vi "Cycle_Time_Test.vi"() -> ()   [LabVIEW 2017]
uses:
  Controls/ADCP_UI/ADCP_UI_Data_Packet_Receiver_Parameters.ctl
  Controls/Connection Management/Connection_Management_Commands.ctl
  Controls/Packet/Packet.ctl
  Controls/Packet/Packet_Direction.ctl
  Controls/Packet/Packet_Type.ctl
  Controls/Packet/Packet_Priority.ctl
  <vilib>/Instr/_visa.llb/VISA Flush IO Buffer Mask.ctl
panel:
  in  "Node ID":u8
  in  "Stop":bool
  out "Received Packet Data":T1[](array[typedef])
  in  "baud rate":u32=9600
  in  "COM Port In":refnum<visa-resource-name>
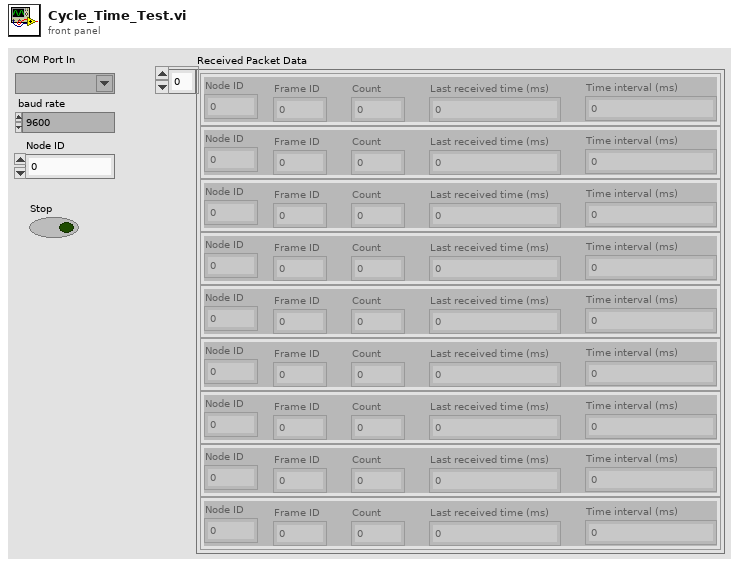
[diagram p1: front panel]
types:
  T1 = typedef "ADCP_UI_Data_Packet_Receiver_Parameters.ctl" = cluster{"Node ID":u32, "Frame ID":u32, "Count":u32, "Last received time (ms)":u32, "Time interval (ms)":u32}
  T2 = typedef "Packet.ctl" = cluster{"Raw Bytes":u8[], "Checksum":bool, "Direction":T3, "Processed Bytes":u8[], "Node ID":u8, "Packet type":T4, "Frame Data":u32, "Priority":T5, "Frame ID":u8}
  T3 = typedef "Packet_Direction.ctl" = enum16{"Transmit", "Receive", "Bidirectional"}
  T4 = typedef "Packet_Type.ctl" = enum16{"Data", "Connection Management", "Remote Request", "Error/Status"}
  T5 = typedef "Packet_Priority.ctl" = enum16{"LOW", "HIGH"}
  T6 = typedef "Connection_Management_Commands.ctl" = enum16{"Sync/Reset", "Open Connection", "Close Connection"}
  T7 = typedef "VISA Flush IO Buffer Mask.ctl" = u16
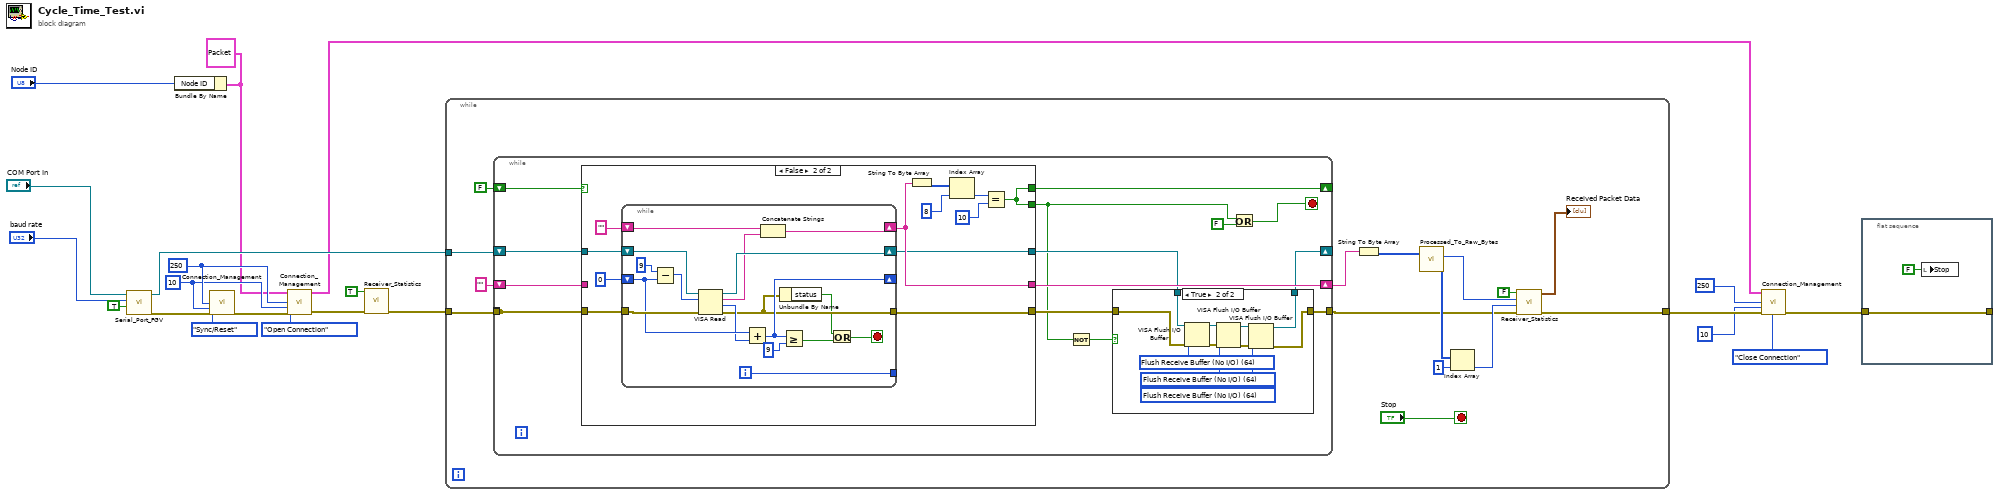
[diagram p0: block diagram]
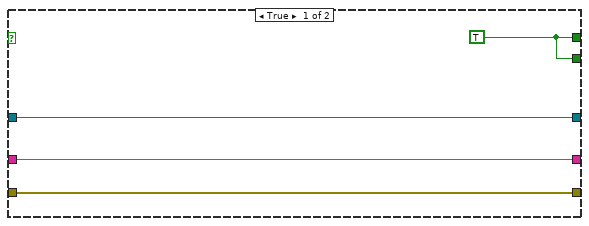
[diagram p3: hidden frame]
diagram:
  w3 = T2 {"Raw Bytes"=[], "Checksum"=FALSE, "Direction"=enum."Transmit", "Processed Bytes"=[], "Node ID"=0, "Packet type"=enum."Data", "Frame Data"=0, "Priority"=enum."LOW", "Frame ID"=0} ("CM Packet In")
  w14 = u8 10 ("Number of tries")
  w15 = 250 ("Retry interval (ms)")
  n1 = call "Serial_Port_FGV.vi"("Initialize ?"=TRUE, "baud rate"="baud rate", "COM Port In"="COM Port In") -> ("error out"=w18:errorcluster, "COM Port out"=w12:refnum<visa-resource-name>)  [unwired: 7 in]
  n2 = Bundle By Name(cluster=w3, "Node ID"="Node ID") -> ()  [unwired: 1 out]
  n3 = call "Connection_Management.vi"("Commands"=Connection_Management_Commands."Sync/Reset", "Retry interval (ms)"=w15, "Number of tries"=w14, "error in (no error)"=w18) -> ("error out"=w16:errorcluster)  [unwired: 8 in, 3 out]
  n4 = call "Connection_Management.vi"("CM Packet In"=w3, "Commands"=Connection_Management_Commands."Open Connection", "Retry interval (ms)"=w15, "Number of tries"=w14, "error in (no error)"=w16) -> ("CM Packet Out"=w1:T2, "error out"=w5:errorcluster)  [unwired: 7 in, 2 out]
  n5 = call "Receiver_Statistics.vi"("error in (no error)"=w5, "Initialize ?"=TRUE) -> ("error out"=w4:errorcluster)  [unwired: 7 in, 2 out]
  n6 = while {
    tunnel: w12 -> [w34]
    tunnel: w4 -> [w33]
    tunnel: [w22] -> w10
    stop <- "Stop" stop-if-true
    n7 = while {
      tunnel: w33 -> [w45]
      shift-right: [w48] -> _
      shift-left: FALSE -> [w49]
      tunnel: [w43] -> w23
      shift-right: [w47] -> w31
      shift-left: "" -> [w46]
      shift-right: [w41] -> _
      shift-left: w34 -> [w50]
      tunnel: [w45] -> _
      stop <- w40 stop-if-true
      n8 = case shown="False" w49 {
        tunnel: w45 -> [w66 w79]
        tunnel: w50 -> [w64 w77]
        tunnel: [w67 w71] -> w38
        tunnel: [w67 w71] -> w48
        tunnel: [w66 w70] -> w44
        tunnel: [w65 w69] -> w47
        tunnel: w46 -> [w65 _]
        tunnel: [w64 w68] -> w42
        frame True {
          w67 = TRUE
        }
        frame False {
          n9 = while {
            tunnel: w79 -> [w96]
            shift-right: [w86] -> _
            shift-left: 0 -> [w89]
            shift-right: [w92] -> w68
            shift-left: w77 -> [w93]
            shift-right: [w85] -> w69
            shift-left: "" -> [w91]
            tunnel: [w81] -> w70
            tunnel: [w84] -> _
            i -> [w84]
            stop <- w83 stop-if-true
            n10 = Subtract(x=9, y=w89) -> (x-y=w94:u32)
            n11 = VISA Read(VISA resource name=w93, byte count=w94, error in (no error)=w96) -> (VISA resource name out=w92:refnum<visa-resource-name>, read buffer=w90:string, return count=w88:u32, error out=w81:errorcluster)
            n12 = Add(x=w89, y=w88) -> (x+y=w86:u32)
            n13 = Concatenate Strings(w91, w90) -> (w85:string)
            n14 = Unbundle By Name(w81) -> ("status"=w80:bool)
            n15 = Greater Or Equal?(x=w86, y=u32 9) -> (x >= y?=w82:bool)
            n16 = Or(x=w80, y=w82) -> (x .or. y?=w83:bool)
          }
          n17 = String To Byte Array(string=w69) -> (unsigned byte array=w75:u8[])
          n18 = Index Array(array=w75, index=8) -> (element=w73:u8)
          n19 = Equal?(x=w73, y=u8 10) -> (x = y?=w71:bool)
        }
      }
      n20 = Not(x=w38) -> (.not. x?=w37:bool)
      n21 = case shown="True" w37 {
        tunnel: w44 -> [w52 w63]
        tunnel: [w52 w60] -> w43
        tunnel: w42 -> [w51 w59]
        tunnel: [w51 w56] -> w41
        frame False {
        }
        frame True {
          w53 = T7 64 items=["Flush Receive Buffer"=16, "Write Transmit Buffer to Device"=32, "Flush Receive Buffer (No I/O)"=64, "Flush Transmit Buffer"=128] ("Mask")
          w54 = T7 64 items=["Flush Receive Buffer"=16, "Write Transmit Buffer to Device"=32, "Flush Receive Buffer (No I/O)"=64, "Flush Transmit Buffer"=128] ("Mask")
          w55 = T7 64 items=["Flush Receive Buffer"=16, "Write Transmit Buffer to Device"=32, "Flush Receive Buffer (No I/O)"=64, "Flush Transmit Buffer"=128] ("Mask")
          n22 = VISA Flush I/O Buffer(VISA resource name=w59, mask (16)=w55, error in (no error)=w63) -> (VISA resource name out=w58:refnum<visa-resource-name>, error out=w62:errorcluster)
          n23 = VISA Flush I/O Buffer(VISA resource name=w58, mask (16)=w54, error in (no error)=w62) -> (VISA resource name out=w57:refnum<visa-resource-name>, error out=w61:errorcluster)
          n24 = VISA Flush I/O Buffer(VISA resource name=w57, mask (16)=w53, error in (no error)=w61) -> (VISA resource name out=w56:refnum<visa-resource-name>, error out=w60:errorcluster)
        }
      }
      n25 = Or(x=w38, y=FALSE) -> (x .or. y?=w40:bool)
    }
    n26 = String To Byte Array(string=w31) -> (unsigned byte array=w32:u8[])
    n27 = call "Processed_To_Raw_Bytes.vi"("Processed Bytes"=w32) -> ("Node ID"=w30:u8, "Raw Bytes"=w29:u8[])  [unwired: 1 in, 3 out]
    n28 = Index Array(array=w29, index=1) -> (element=w27:u8)
    n29 = call "Receiver_Statistics.vi"("error in (no error)"=w23, "Frame ID"=w27, "Node ID"=w30, "Initialize ?"=FALSE) -> ("error out"=w22:errorcluster, "Received Packet Data"=→"Received Packet Data":T1[])  [unwired: 5 in, 1 out]
  }
  n30 = call "Connection_Management.vi"("CM Packet In"=w1, "Commands"=Connection_Management_Commands."Close Connection", "Retry interval (ms)"=250, "Number of tries"=u8 10, "error in (no error)"=w10) -> ("error out"=w6:errorcluster)  [unwired: 7 in, 3 out]
  n31 = flat-sequence {
    tunnel: w6 -> [w98]
    tunnel: [w98] -> _
    frame #0 {
      n32 = local write "Stop"(FALSE ("Stop")) -> ()
    }
  }
